vi "Teardown.vi"(11 "Queue Transport in":refnum<class "Queue Transport.lvclass">) -> (2 "Unhandled Msgs":refnum<class "Msg.lvclass">[](array[class]))   [LabVIEW 2025, in "jettl.lvlib" / "Transport.lvlib" / "Queue Transport.lvclass"]
uses:
  Queue Transport.lvclass
  Queue Transport.lvclass/Queue Transport.ctl
  Msg/Msg.lvclass
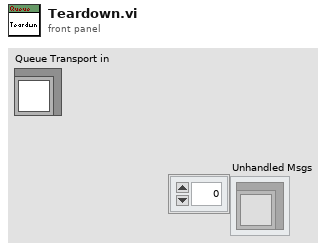
[diagram p1: front panel]
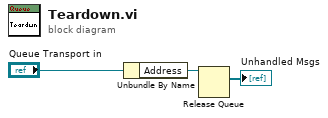
[diagram p0: block diagram]
diagram:
  n1 = Unbundle By Name("Queue Transport in") -> ("Address"=w2:refnum<queue>)
  n2 = Release Queue(queue=w2) -> (remaining elements=→"Unhandled Msgs":refnum<class "Msg.lvclass">[])  [unwired: 2 in, 2 out]
